vi "dfd_LatticeARMA_Basic_IIR_C.vi"() -> ()   [LabVIEW 2017, in "NI_DigFilterTemp.lvlib"]
uses:
  <vilib>/addons/Digital Filter Design/NI_DigFilterTemp.lvlib
panel:
  in  "String":string="\n\n/* ---- Constants ----*/\n#define %CapName%_N_COEFK %kIIRStatesAmt%\n#define %CapName%_N_COEFV (%CapName%_N_COEFK + 1)\n#define %CapName%_N_STATES %CapName%_N_COEFV\n\n/* ---- Global Variables Declaration ----*/\nstatic %CoefAType% %FilterBlkName%_CoefK[%CapName%_N_COEFK];\nstatic %CoefBType% %FilterBlkName%_CoefV[%CapName%_N_COEFV];\n%InternalFunctionsDeclaration%\n\n%ShiftDefine%\n\n%AssistantFunctions%\n\n/* ---- Implement the Fixed-Point Filter ---- */ \n%OutType% %FilterBlkName%_Filtering (%InType% sampleIn, %FilterBlkName%_State state)\n{\n\tI32 accA, accB, accTmp;\n\t%MultType% mult;\n\tint i;\n\t\n\taccB = (%I32TypeCast%sampleIn << IN2SUM);\n\n\t/* Filtering */\n\tfor (i=0; i < %CapName%_N_COEFK; i++)\n\t{\n\t\tmult = %PreMultCast%(state[i] << DELAY2MULT);\n\t\taccB -= (%FilterBlkName%_%MultA%(mult, %FilterBlkName%_CoefK[i]) << PROD2SUM);\n\t\tmult = %PreMultCast%(accB << SUM2MULT);\n\t\taccA = (%FilterBlkName%_%MultA%(mult, %FilterBlkName%_CoefK[i]) << PROD2SUM);\n\t\taccA += (state[i] << DELAY2SUM);\n\t\tstate[i] = accA;\n\t}\n\t\n\taccA = 0;\n\taccTmp = 0;\n\n\t/* Filtering and update the internal states */\n\tfor (i=%CapName%_N_COEFV-1; i >= 0; i--)\n\t{\n\t\tstate[i] = (accTmp << SUM2DELAY);\n\t\tmult = %PreMultCast%(accB << SUM2MULT);\n\t\taccA += (%FilterBlkName%_%MultB%(mult, %FilterBlkName%_CoefV[i]) << PROD2SUM);\n\t\taccTmp = accB;\n\t\taccB = (i==0) ? 0 : state[i-1];\n\t}\n\n\t%ApplyGainAccA%\n\n\treturn (%OutType%)accA;\n}\n\n/* ---- Internal Functions ---- */\n%InternalFunctions%\n\n/* ---- Filter Coefficients ---- */\nstatic %CoefAType% %FilterBlkName%_CoefK [] = {\n%CoefficientsK%\n};\nstatic %CoefBType% %FilterBlkName%_CoefV [] = {\n%CoefficientsV%\n};\n"
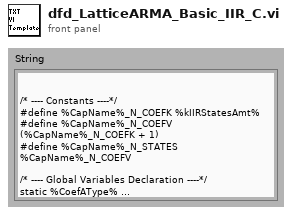
[diagram p1: front panel]
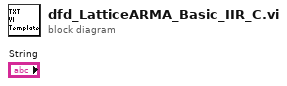
[diagram p0: block diagram]
diagram:
